vi "总氮单步调试对话框.vi"() -> ()   [LabVIEW 2016, in "斯坦道总氮.lvlib"]
panel:
  in  "停止":bool
  out "温度2":sgl
  out "温度1":sgl
  out "ADC":sgl
  out "F3":sgl format="%#.6f"
  out "F2":sgl format="%#.6f"
  out "F1":sgl format="%#.6f"
  out "F0":sgl format="%#.6f"
  in  "退出":bool
  in  "启动":bool
  in  "总磷氨氮调试":u16[](xcontrol)
  # "总氮单步调试界面"
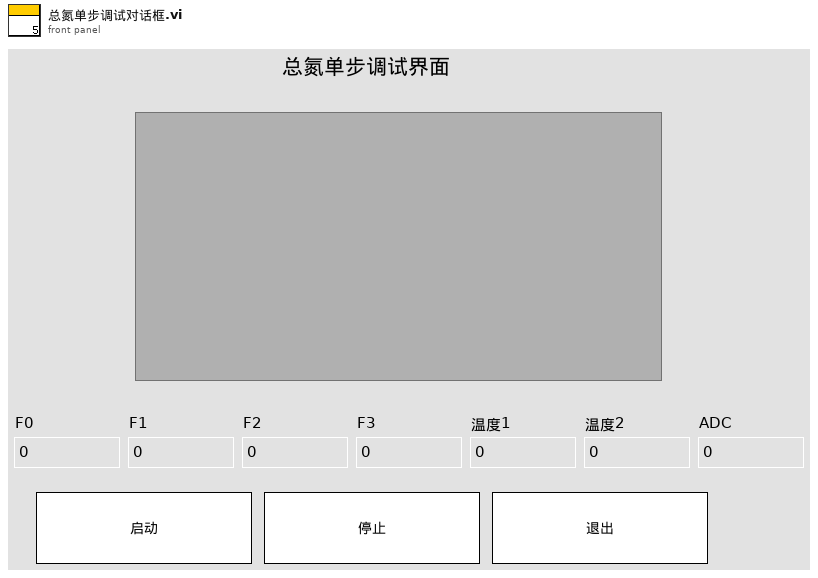
[diagram p1: front panel]
types:
  T1 = cluster{"阀口名称自定义类型":enum16{"自定义", "微站总磷总氮", "微站总磷氨氮", "微站氨氮", "固定站总磷", "固定站总氮", "固定站氨氮", "原位总磷总氮", "原位总磷氨氮", "原位总磷", "原位总氮", "原位氨氮", "原位3N1P"}, "阀口自定义名称":cluster{"V1":string, "V2":string, "V3":string, "V4":string, "V5":string, "V6":string, "V7":string, "V8":string, "V9":string, "V10":string, "V11":string, "V12":string, "V9-1":string, "V9-2":string}}
  T2 = enum16{"自定义", "微站总磷总氮", "微站总磷氨氮", "微站氨氮", "固定站总磷", "固定站总氮", "固定站氨氮", "原位总磷总氮", "原位总磷氨氮", "原位总磷", "原位总氮", "原位氨氮", "原位3N1P"}
  T3 = cluster{"系统时间":timestamp, "工作状态":enum16{"空闲", "水样测试", "标样核查", "零点核查", "跨度核查", "空白测试", "平行样测试", "加标回收", "空白校准", "标样校准", "初始化（清洗）"}, "测量模式":enum16{"待机", "连续模式", "周期模式", "定点模式", "受控模式", "手动模式"}, "告警代码":u16, "故障代码":u16, "日志代码":u16, "软件版本":u16, "F0":sgl, "F1":sgl, "F2":sgl, "F3":sgl, "T":sgl, "H":sgl, "id":u16, "flowid":u16, "量程":u16, "总磷控温温度1":sgl, "营养盐控温温度2":sgl, "ADC":sgl}
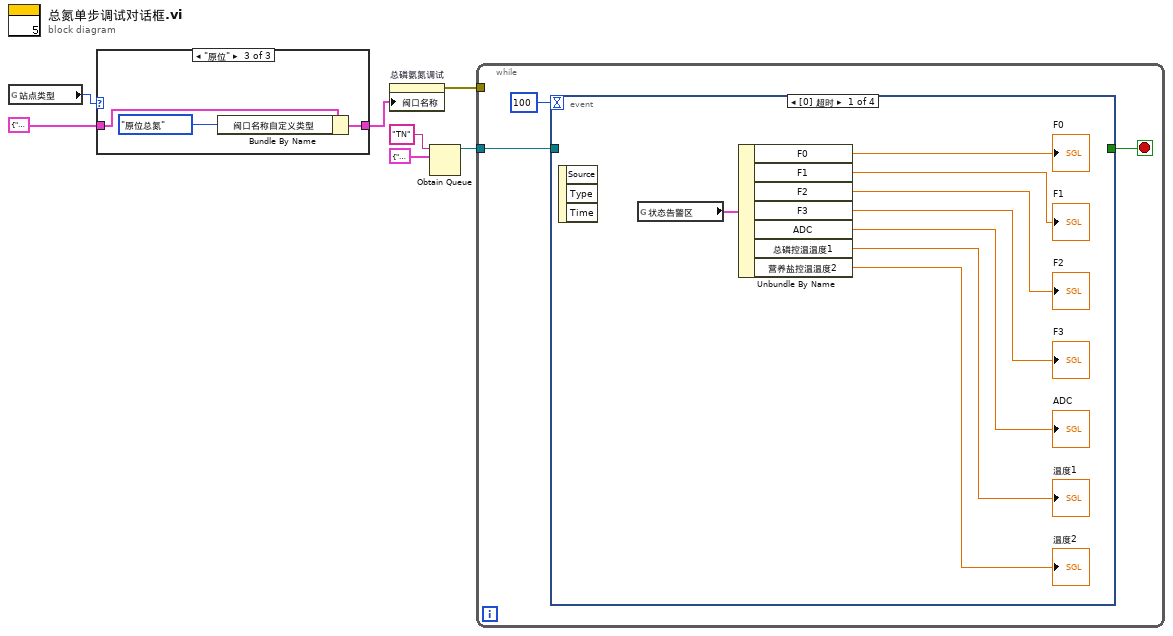
[diagram p0: block diagram]
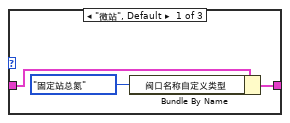
[diagram p2: hidden frame]
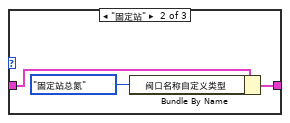
[diagram p3: hidden frame]
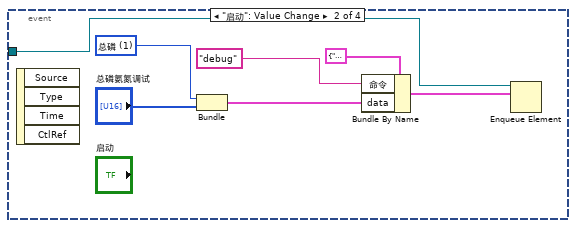
[diagram p4: hidden frame]
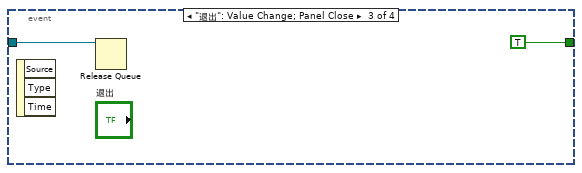
[diagram p5: hidden frame]
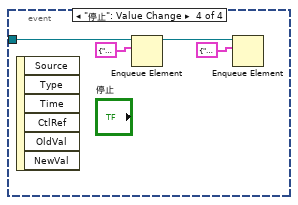
[diagram p6: hidden frame]
diagram:
  n1 = global read "VAR总氮全局变量.vi" "站点类型"() -> (w4:enum16{"微站", "固定站", "原位"})
  n2 = case shown="\"原位\"" w4 {
    tunnel: T1 {"阀口名称自定义类型"=enum."自定义", "阀口自定义名称"={"V1"="", "V2"="", "V3"="", "V4"="", "V5"="", "V6"="", "V7"="", "V8"="", "V9"="", "V10"="", "V11"="", "V12"="", "V9-1"="", "V9-2"=""}} ("阀口名称") -> [w10 w13 w16]
    tunnel: [w9 w12 w15] -> w1
    frame "微站", Default {
      n3 = Bundle By Name(cluster=w10, "阀口名称自定义类型"=T2."固定站总氮") -> (w9:T1)
    }
    frame "固定站" {
      n4 = Bundle By Name(cluster=w13, "阀口名称自定义类型"=T2."固定站总氮") -> (w12:T1)
    }
    frame "原位" {
      n5 = Bundle By Name(cluster=w16, "阀口名称自定义类型"=T2."原位总氮") -> (w15:T1)
    }
  }
  n6 = property on="总磷氨氮调试" class="调试控件V3 (严格)"("阀口名称"=w1) -> (error out=w3:errorcluster)  [unwired: 2 in, 1 out]
  n7 = Obtain Queue(name (unnamed)="TN" ("名称（未命名）"), element data type=cluster{"命令":string, "data":variant} {"命令"="", "data"=variant}) -> (queue out=w5:refnum<queue>)  [unwired: 3 in, 2 out]
  n8 = while {
    tunnel: w5 -> [w19]
    tunnel: w3 -> [_]
    stop <- w18 stop-if-true
    n9 = event shown="[0] 超时" {
      selector: _ -> [_ _ _ _]
      dyn-events: _ -> [_ _ _ _]
      timeout: 100 -> [_ _ _ _]
      tunnel: w19 -> [_ w29 w35 w37]
      tunnel: [_ _ TRUE _] -> w18
      event Timeout {
        n10 = event-data() -> ()  [unwired: 1 in, 3 out]
        n11 = global read "VAR总氮全局变量.vi" "状态告警区"() -> (w27:T3)
        n12 = Unbundle By Name(w27) -> ("F0"=→"F0":sgl, "F1"=→"F1":sgl, "F2"=→"F2":sgl, "F3"=→"F3":sgl, "ADC"=→"ADC":sgl, "总磷控温温度1"=→"温度1":sgl, "营养盐控温温度2"=→"温度2":sgl)
      }
      event "启动": Value Change {
        w31 = u16 1 items=["总磷"=1, "氨氮"=3] ("站号")
        n13 = event-data() -> ()  [unwired: 1 in, 4 out]
        n14 = Bundle("站号"=w31, "总磷氨氮调试"="总磷氨氮调试") -> (w30:cluster{"站号":u16, "总磷氨氮调试":u16[]})  [unwired: 1 in]
        n15 = Bundle By Name(cluster=cluster{"命令":string, "data":variant} {"命令"="", "data"=variant} ("元素"), "命令"="debug", "data"=w30) -> (w32:cluster{"命令":string, "data":variant})
        n16 = Enqueue Element(queue=w29, element=w32) -> ()  [unwired: 2 in, 3 out]
      }
      event "退出": Value Change; Panel Close {
        n17 = event-data() -> ()  [unwired: 1 in, 3 out]
        n18 = Release Queue(queue=w35) -> ()  [unwired: 2 in, 3 out]
      }
      event "停止": Value Change {
        n19 = event-data() -> ()  [unwired: 1 in, 6 out]
        n20 = Enqueue Element(queue=w37, element=cluster{"命令":string, "data":variant} {"命令"="启动", "data"=variant(cluster{"站号":u16, "控制命令输出":u16[]} {"站号"=1, "控制命令输出"=[2816]})} ("元素")) -> (queue out=w38:refnum<queue>)  [unwired: 2 in, 2 out]
        n21 = Enqueue Element(queue=w38, element=cluster{"命令":string, "data":variant} {"命令"="启动", "data"=variant(cluster{"站号":u16, "控制命令输出":u16[]} {"站号"=2, "控制命令输出"=[2816]})} ("元素")) -> ()  [unwired: 2 in, 3 out]
      }
    }
  }
